vi "Array Variant to Cluster Variant.vi"(1 "Array":variant[](array[variant])) -> (0 "Cluster":variant)   [LabVIEW 2017, in "LabPack.lvlib"] (continued)
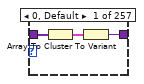
[diagram p2: hidden frame]
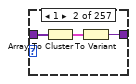
[diagram p3: hidden frame]
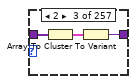
[diagram p4: hidden frame]
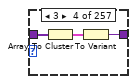
[diagram p5: hidden frame]
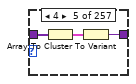
[diagram p6: hidden frame]
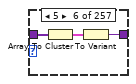
[diagram p7: hidden frame]
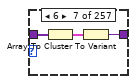
[diagram p8: hidden frame]
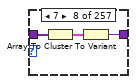
[diagram p9: hidden frame]
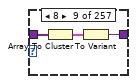
[diagram p10: hidden frame]
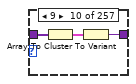
[diagram p11: hidden frame]
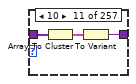
[diagram p12: hidden frame]
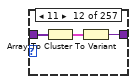
[diagram p13: hidden frame]
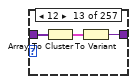
[diagram p14: hidden frame]
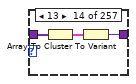
[diagram p15: hidden frame]
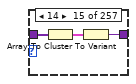
[diagram p16: hidden frame]
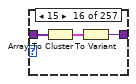
[diagram p17: hidden frame]
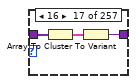
[diagram p18: hidden frame]
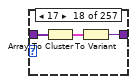
[diagram p19: hidden frame]
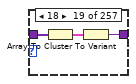
[diagram p20: hidden frame]
      n45 = Array To Cluster(array=w69) -> (cluster=w68:T19)
      n46 = To Variant(anything=w68) -> (Variant=w67:variant)
    }
    frame 22 {
      n47 = Array To Cluster(array=w72) -> (cluster=w71:T20)
      n48 = To Variant(anything=w71) -> (Variant=w70:variant)
    }
    frame 23 {
      n49 = Array To Cluster(array=w75) -> (cluster=w74:T21)
      n50 = To Variant(anything=w74) -> (Variant=w73:variant)
    }
    frame 24 {
      n51 = Array To Cluster(array=w78) -> (cluster=w77:T22)
      n52 = To Variant(anything=w77) -> (Variant=w76:variant)
    }
    frame 25 {
      n53 = Array To Cluster(array=w81) -> (cluster=w80:T23)
      n54 = To Variant(anything=w80) -> (Variant=w79:variant)
    }
    frame 26 {
      n55 = Array To Cluster(array=w84) -> (cluster=w83:T24)
      n56 = To Variant(anything=w83) -> (Variant=w82:variant)
    }
    frame 27 {
      n57 = Array To Cluster(array=w87) -> (cluster=w86:T25)
      n58 = To Variant(anything=w86) -> (Variant=w85:variant)
    }
    frame 28 {
      n59 = Array To Cluster(array=w90) -> (cluster=w89:T26)
      n60 = To Variant(anything=w89) -> (Variant=w88:variant)
    }
    frame 29 {
      n61 = Array To Cluster(array=w93) -> (cluster=w92:T27)
      n62 = To Variant(anything=w92) -> (Variant=w91:variant)
    }
    frame 30 {
      n63 = Array To Cluster(array=w96) -> (cluster=w95:T28)
      n64 = To Variant(anything=w95) -> (Variant=w94:variant)
    }
    frame 31 {
      n65 = Array To Cluster(array=w99) -> (cluster=w98:T29)
      n66 = To Variant(anything=w98) -> (Variant=w97:variant)
    }
    frame 32 {
      n67 = Array To Cluster(array=w102) -> (cluster=w101:T30)
      n68 = To Variant(anything=w101) -> (Variant=w100:variant)
    }
    frame 33 {
      n69 = Array To Cluster(array=w105) -> (cluster=w104:T31)
      n70 = To Variant(anything=w104) -> (Variant=w103:variant)
    }
    frame 34 {
      n71 = Array To Cluster(array=w108) -> (cluster=w107:T32)
      n72 = To Variant(anything=w107) -> (Variant=w106:variant)
    }
    frame 35 {
      n73 = Array To Cluster(array=w111) -> (cluster=w110:T33)
      n74 = To Variant(anything=w110) -> (Variant=w109:variant)
    }
    frame 36 {
      n75 = Array To Cluster(array=w114) -> (cluster=w113:T34)
      n76 = To Variant(anything=w113) -> (Variant=w112:variant)
    }
    frame 37 {
      n77 = Array To Cluster(array=w117) -> (cluster=w116:T35)
      n78 = To Variant(anything=w116) -> (Variant=w115:variant)
    }
    frame 38 {
      n79 = Array To Cluster(array=w120) -> (cluster=w119:T36)
      n80 = To Variant(anything=w119) -> (Variant=w118:variant)
    }
    frame 39 {
      n81 = Array To Cluster(array=w123) -> (cluster=w122:T37)
      n82 = To Variant(anything=w122) -> (Variant=w121:variant)
    }
    frame 40 {
      n83 = Array To Cluster(array=w126) -> (cluster=w125:T38)
      n84 = To Variant(anything=w125) -> (Variant=w124:variant)
    }
    frame 41 {
      n85 = Array To Cluster(array=w129) -> (cluster=w128:T39)
      n86 = To Variant(anything=w128) -> (Variant=w127:variant)
    }
    frame 42 {
      n87 = Array To Cluster(array=w132) -> (cluster=w131:T40)
      n88 = To Variant(anything=w131) -> (Variant=w130:variant)
    }
    frame 43 {
      n89 = Array To Cluster(array=w135) -> (cluster=w134:T41)
      n90 = To Variant(anything=w134) -> (Variant=w133:variant)
    }
    frame 44 {
      n91 = Array To Cluster(array=w138) -> (cluster=w137:T42)
      n92 = To Variant(anything=w137) -> (Variant=w136:variant)
    }
    frame 45 {
      n93 = Array To Cluster(array=w141) -> (cluster=w140:T43)
      n94 = To Variant(anything=w140) -> (Variant=w139:variant)
    }
    frame 46 {
      n95 = Array To Cluster(array=w144) -> (cluster=w143:T44)
      n96 = To Variant(anything=w143) -> (Variant=w142:variant)
    }
    frame 47 {
      n97 = Array To Cluster(array=w147) -> (cluster=w146:T45)
      n98 = To Variant(anything=w146) -> (Variant=w145:variant)
    }
    frame 48 {
      n99 = Array To Cluster(array=w150) -> (cluster=w149:T46)
      n100 = To Variant(anything=w149) -> (Variant=w148:variant)
    }
    frame 49 {
      n101 = Array To Cluster(array=w153) -> (cluster=w152:T47)
      n102 = To Variant(anything=w152) -> (Variant=w151:variant)
    }
    frame 50 {
      n103 = Array To Cluster(array=w156) -> (cluster=w155:T48)
      n104 = To Variant(anything=w155) -> (Variant=w154:variant)
    }
    frame 51 {
      n105 = Array To Cluster(array=w159) -> (cluster=w158:T49)
      n106 = To Variant(anything=w158) -> (Variant=w157:variant)
    }
    frame 52 {
      n107 = Array To Cluster(array=w162) -> (cluster=w161:T50)
      n108 = To Variant(anything=w161) -> (Variant=w160:variant)
    }
    frame 53 {
      n109 = Array To Cluster(array=w165) -> (cluster=w164:T51)
      n110 = To Variant(anything=w164) -> (Variant=w163:variant)
    }
    frame 54 {
      n111 = Array To Cluster(array=w168) -> (cluster=w167:T52)
      n112 = To Variant(anything=w167) -> (Variant=w166:variant)
    }
    frame 55 {
      n113 = Array To Cluster(array=w171) -> (cluster=w170:T53)
      n114 = To Variant(anything=w170) -> (Variant=w169:variant)
    }
    frame 56 {
      n115 = Array To Cluster(array=w174) -> (cluster=w173:T54)
      n116 = To Variant(anything=w173) -> (Variant=w172:variant)
    }
    frame 57 {
      n117 = Array To Cluster(array=w177) -> (cluster=w176:T55)
      n118 = To Variant(anything=w176) -> (Variant=w175:variant)
    }
    frame 58 {
      n119 = Array To Cluster(array=w180) -> (cluster=w179:T56)
      n120 = To Variant(anything=w179) -> (Variant=w178:variant)
    }
    frame 59 {
      n121 = Array To Cluster(array=w183) -> (cluster=w182:T57)
      n122 = To Variant(anything=w182) -> (Variant=w181:variant)
    }
    frame 60 {
      n123 = Array To Cluster(array=w186) -> (cluster=w185:T58)
      n124 = To Variant(anything=w185) -> (Variant=w184:variant)
    }
    frame 61 {
      n125 = Array To Cluster(array=w189) -> (cluster=w188:T59)
      n126 = To Variant(anything=w188) -> (Variant=w187:variant)
    }
    frame 62 {
      n127 = Array To Cluster(array=w192) -> (cluster=w191:T60)
      n128 = To Variant(anything=w191) -> (Variant=w190:variant)
    }
    frame 63 {
      n129 = Array To Cluster(array=w195) -> (cluster=w194:T61)
      n130 = To Variant(anything=w194) -> (Variant=w193:variant)
    }
    frame 64 {
      n131 = Array To Cluster(array=w198) -> (cluster=w197:T62)
      n132 = To Variant(anything=w197) -> (Variant=w196:variant)
    }
    frame 65 {
      n133 = Array To Cluster(array=w201) -> (cluster=w200:T63)
      n134 = To Variant(anything=w200) -> (Variant=w199:variant)
    }
    frame 66 {
      n135 = Array To Cluster(array=w204) -> (cluster=w203:T64)
      n136 = To Variant(anything=w203) -> (Variant=w202:variant)
    }
    frame 67 {
      n137 = Array To Cluster(array=w207) -> (cluster=w206:T65)
      n138 = To Variant(anything=w206) -> (Variant=w205:variant)
    }
    frame 68 {
      n139 = Array To Cluster(array=w210) -> (cluster=w209:T66)
      n140 = To Variant(anything=w209) -> (Variant=w208:variant)
    }
    frame 69 {
      n141 = Array To Cluster(array=w213) -> (cluster=w212:T67)
      n142 = To Variant(anything=w212) -> (Variant=w211:variant)
    }
    frame 70 {
      n143 = Array To Cluster(array=w216) -> (cluster=w215:T68)
      n144 = To Variant(anything=w215) -> (Variant=w214:variant)
    }
    frame 71 {
      n145 = Array To Cluster(array=w219) -> (cluster=w218:T69)
      n146 = To Variant(anything=w218) -> (Variant=w217:variant)
    }
    frame 72 {
      n147 = Array To Cluster(array=w222) -> (cluster=w221:T70)
      n148 = To Variant(anything=w221) -> (Variant=w220:variant)
    }
    frame 73 {
      n149 = Array To Cluster(array=w225) -> (cluster=w224:T71)
      n150 = To Variant(anything=w224) -> (Variant=w223:variant)
    }
    frame 74 {
      n151 = Array To Cluster(array=w228) -> (cluster=w227:T72)
      n152 = To Variant(anything=w227) -> (Variant=w226:variant)
    }
    frame 75 {
      n153 = Array To Cluster(array=w231) -> (cluster=w230:T73)
      n154 = To Variant(anything=w230) -> (Variant=w229:variant)
    }
    frame 76 {
      n155 = Array To Cluster(array=w234) -> (cluster=w233:T74)
      n156 = To Variant(anything=w233) -> (Variant=w232:variant)
    }
    frame 77 {
      n157 = Array To Cluster(array=w237) -> (cluster=w236:T75)
      n158 = To Variant(anything=w236) -> (Variant=w235:variant)
    }
    frame 78 {
      n159 = Array To Cluster(array=w240) -> (cluster=w239:T76)
      n160 = To Variant(anything=w239) -> (Variant=w238:variant)
    }
    frame 79 {
      n161 = Array To Cluster(array=w243) -> (cluster=w242:T77)
      n162 = To Variant(anything=w242) -> (Variant=w241:variant)
    }
    frame 80 {
      n163 = Array To Cluster(array=w246) -> (cluster=w245:T78)
      n164 = To Variant(anything=w245) -> (Variant=w244:variant)
    }
    frame 81 {
      n165 = Array To Cluster(array=w249) -> (cluster=w248:T79)
      n166 = To Variant(anything=w248) -> (Variant=w247:variant)
    }
    frame 82 {
      n167 = Array To Cluster(array=w252) -> (cluster=w251:T80)
      n168 = To Variant(anything=w251) -> (Variant=w250:variant)
    }
    frame 83 {
      n169 = Array To Cluster(array=w255) -> (cluster=w254:T81)
      n170 = To Variant(anything=w254) -> (Variant=w253:variant)
    }
    frame 84 {
      n171 = Array To Cluster(array=w258) -> (cluster=w257:T82)
      n172 = To Variant(anything=w257) -> (Variant=w256:variant)
    }
    frame 85 {
      n173 = Array To Cluster(array=w261) -> (cluster=w260:T83)
      n174 = To Variant(anything=w260) -> (Variant=w259:variant)
    }
    frame 86 {
      n175 = Array To Cluster(array=w264) -> (cluster=w263:T84)
      n176 = To Variant(anything=w263) -> (Variant=w262:variant)
    }
    frame 87 {
      n177 = Array To Cluster(array=w267) -> (cluster=w266:T85)
      n178 = To Variant(anything=w266) -> (Variant=w265:variant)
    }
    frame 88 {
      n179 = Array To Cluster(array=w270) -> (cluster=w269:T86)
      n180 = To Variant(anything=w269) -> (Variant=w268:variant)
    }
    frame 89 {
      n181 = Array To Cluster(array=w273) -> (cluster=w272:T87)
      n182 = To Variant(anything=w272) -> (Variant=w271:variant)
    }
    frame 90 {
      n183 = Array To Cluster(array=w276) -> (cluster=w275:T88)
      n184 = To Variant(anything=w275) -> (Variant=w274:variant)
    }
    frame 91 {
      n185 = Array To Cluster(array=w279) -> (cluster=w278:T89)
      n186 = To Variant(anything=w278) -> (Variant=w277:variant)
    }
    frame 92 {
      n187 = Array To Cluster(array=w282) -> (cluster=w281:T90)
      n188 = To Variant(anything=w281) -> (Variant=w280:variant)
    }
    frame 93 {
      n189 = Array To Cluster(array=w285) -> (cluster=w284:T91)
      n190 = To Variant(anything=w284) -> (Variant=w283:variant)
    }
    frame 94 {
      n191 = Array To Cluster(array=w288) -> (cluster=w287:T92)
      n192 = To Variant(anything=w287) -> (Variant=w286:variant)
    }
    frame 95 {
      n193 = Array To Cluster(array=w291) -> (cluster=w290:T93)
      n194 = To Variant(anything=w290) -> (Variant=w289:variant)
    }
    frame 96 {
      n195 = Array To Cluster(array=w294) -> (cluster=w293:T94)
      n196 = To Variant(anything=w293) -> (Variant=w292:variant)
    }
    frame 97 {
      n197 = Array To Cluster(array=w297) -> (cluster=w296:T95)
      n198 = To Variant(anything=w296) -> (Variant=w295:variant)
    }
    frame 98 {
      n199 = Array To Cluster(array=w300) -> (cluster=w299:T96)
      n200 = To Variant(anything=w299) -> (Variant=w298:variant)
    }
    frame 99 {
      n201 = Array To Cluster(array=w303) -> (cluster=w302:T97)
      n202 = To Variant(anything=w302) -> (Variant=w301:variant)
    }
    frame 100 {
      n203 = Array To Cluster(array=w306) -> (cluster=w305:T98)
      n204 = To Variant(anything=w305) -> (Variant=w304:variant)
    }
    frame 101 {
      n205 = Array To Cluster(array=w309) -> (cluster=w308:T99)
      n206 = To Variant(anything=w308) -> (Variant=w307:variant)
    }
    frame 102 {
      n207 = Array To Cluster(array=w312) -> (cluster=w311:T100)
      n208 = To Variant(anything=w311) -> (Variant=w310:variant)
    }
    frame 103 {
      n209 = Array To Cluster(array=w315) -> (cluster=w314:T101)
      n210 = To Variant(anything=w314) -> (Variant=w313:variant)
    }
    frame 104 {
      n211 = Array To Cluster(array=w318) -> (cluster=w317:T102)
      n212 = To Variant(anything=w317) -> (Variant=w316:variant)
    }
    frame 105 {
      n213 = Array To Cluster(array=w321) -> (cluster=w320:T103)
      n214 = To Variant(anything=w320) -> (Variant=w319:variant)
    }
    frame 106 {
      n215 = Array To Cluster(array=w324) -> (cluster=w323:T104)
      n216 = To Variant(anything=w323) -> (Variant=w322:variant)
    }
    frame 107 {
      n217 = Array To Cluster(array=w327) -> (cluster=w326:T105)
      n218 = To Variant(anything=w326) -> (Variant=w325:variant)
    }
    frame 108 {
      n219 = Array To Cluster(array=w330) -> (cluster=w329:T106)
      n220 = To Variant(anything=w329) -> (Variant=w328:variant)
    }
    frame 109 {
      n221 = Array To Cluster(array=w333) -> (cluster=w332:T107)
      n222 = To Variant(anything=w332) -> (Variant=w331:variant)
    }
    frame 110 {
      n223 = Array To Cluster(array=w336) -> (cluster=w335:T108)
      n224 = To Variant(anything=w335) -> (Variant=w334:variant)
    }
    frame 111 {
      n225 = Array To Cluster(array=w339) -> (cluster=w338:T109)
      n226 = To Variant(anything=w338) -> (Variant=w337:variant)
    }
    frame 112 {
      n227 = Array To Cluster(array=w342) -> (cluster=w341:T110)
      n228 = To Variant(anything=w341) -> (Variant=w340:variant)
    }
    frame 113 {
      n229 = Array To Cluster(array=w345) -> (cluster=w344:T111)
      n230 = To Variant(anything=w344) -> (Variant=w343:variant)
    }
    frame 114 {
      n231 = Array To Cluster(array=w348) -> (cluster=w347:T112)
      n232 = To Variant(anything=w347) -> (Variant=w346:variant)
    }
    frame 115 {
      n233 = Array To Cluster(array=w351) -> (cluster=w350:T113)
      n234 = To Variant(anything=w350) -> (Variant=w349:variant)
    }
    frame 116 {
      n235 = Array To Cluster(array=w354) -> (cluster=w353:T114)
      n236 = To Variant(anything=w353) -> (Variant=w352:variant)
    }
    frame 117 {
      n237 = Array To Cluster(array=w357) -> (cluster=w356:T115)
      n238 = To Variant(anything=w356) -> (Variant=w355:variant)
    }
    frame 118 {
      n239 = Array To Cluster(array=w360) -> (cluster=w359:T116)
      n240 = To Variant(anything=w359) -> (Variant=w358:variant)
    }
    frame 119 {
      n241 = Array To Cluster(array=w363) -> (cluster=w362:T117)
      n242 = To Variant(anything=w362) -> (Variant=w361:variant)
    }
    frame 120 {
      n243 = Array To Cluster(array=w366) -> (cluster=w365:T118)
      n244 = To Variant(anything=w365) -> (Variant=w364:variant)
    }
    frame 121 {
      n245 = Array To Cluster(array=w369) -> (cluster=w368:T119)
      n246 = To Variant(anything=w368) -> (Variant=w367:variant)
    }
    frame 122 {
      n247 = Array To Cluster(array=w372) -> (cluster=w371:T120)
      n248 = To Variant(anything=w371) -> (Variant=w370:variant)
    }
    frame 123 {
      n249 = Array To Cluster(array=w375) -> (cluster=w374:T121)
      n250 = To Variant(anything=w374) -> (Variant=w373:variant)
    }
    frame 124 {
      n251 = Array To Cluster(array=w378) -> (cluster=w377:T122)
      n252 = To Variant(anything=w377) -> (Variant=w376:variant)
    }
    frame 125 {
      n253 = Array To Cluster(array=w381) -> (cluster=w380:T123)
      n254 = To Variant(anything=w380) -> (Variant=w379:variant)
    }
    frame 126 {
      n255 = Array To Cluster(array=w384) -> (cluster=w383:T124)
      n256 = To Variant(anything=w383) -> (Variant=w382:variant)
    }
    frame 127 {
      n257 = Array To Cluster(array=w387) -> (cluster=w386:T125)
      n258 = To Variant(anything=w386) -> (Variant=w385:variant)
    }
    frame 128 {
      n259 = Array To Cluster(array=w390) -> (cluster=w389:T126)
      n260 = To Variant(anything=w389) -> (Variant=w388:variant)
    }
    frame 129 {
      n261 = Array To Cluster(array=w393) -> (cluster=w392:T127)
      n262 = To Variant(anything=w392) -> (Variant=w391:variant)
    }
    frame 130 {
      n263 = Array To Cluster(array=w396) -> (cluster=w395:T128)
      n264 = To Variant(anything=w395) -> (Variant=w394:variant)
    }
    frame 131 {
      n265 = Array To Cluster(array=w399) -> (cluster=w398:T129)
      n266 = To Variant(anything=w398) -> (Variant=w397:variant)
    }
    frame 132 {
      n267 = Array To Cluster(array=w402) -> (cluster=w401:T130)
      n268 = To Variant(anything=w401) -> (Variant=w400:variant)
    }
    frame 133 {
      n269 = Array To Cluster(array=w405) -> (cluster=w404:T131)
      n270 = To Variant(anything=w404) -> (Variant=w403:variant)
    }
    frame 134 {
      n271 = Array To Cluster(array=w408) -> (cluster=w407:T132)
      n272 = To Variant(anything=w407) -> (Variant=w406:variant)
    }
    frame 135 {
      n273 = Array To Cluster(array=w411) -> (cluster=w410:T133)
      n274 = To Variant(anything=w410) -> (Variant=w409:variant)
    }
    frame 136 {
      n275 = Array To Cluster(array=w414) -> (cluster=w413:T134)
      n276 = To Variant(anything=w413) -> (Variant=w412:variant)
    }
    frame 137 {
      n277 = Array To Cluster(array=w417) -> (cluster=w416:T135)
      n278 = To Variant(anything=w416) -> (Variant=w415:variant)
    }
    frame 138 {
      n279 = Array To Cluster(array=w420) -> (cluster=w419:T136)
      n280 = To Variant(anything=w419) -> (Variant=w418:variant)
    }
    frame 139 {
      n281 = Array To Cluster(array=w423) -> (cluster=w422:T137)
      n282 = To Variant(anything=w422) -> (Variant=w421:variant)
    }
    frame 140 {
      n283 = Array To Cluster(array=w426) -> (cluster=w425:T138)
      n284 = To Variant(anything=w425) -> (Variant=w424:variant)
    }
    frame 141 {
      n285 = Array To Cluster(array=w429) -> (cluster=w428:T139)
      n286 = To Variant(anything=w428) -> (Variant=w427:variant)
    }
    frame 142 {
      n287 = Array To Cluster(array=w432) -> (cluster=w431:T140)
      n288 = To Variant(anything=w431) -> (Variant=w430:variant)
    }
    frame 143 {
      n289 = Array To Cluster(array=w435) -> (cluster=w434:T141)
      n290 = To Variant(anything=w434) -> (Variant=w433:variant)
    }
    frame 144 {
      n291 = Array To Cluster(array=w438) -> (cluster=w437:T142)
      n292 = To Variant(anything=w437) -> (Variant=w436:variant)
    }
    frame 145 {
      n293 = Array To Cluster(array=w441) -> (cluster=w440:T143)
      n294 = To Variant(anything=w440) -> (Variant=w439:variant)
    }
    frame 146 {
      n295 = Array To Cluster(array=w444) -> (cluster=w443:T144)
      n296 = To Variant(anything=w443) -> (Variant=w442:variant)
    }
    frame 147 {
      n297 = Array To Cluster(array=w447) -> (cluster=w446:T145)
      n298 = To Variant(anything=w446) -> (Variant=w445:variant)
    }
    frame 148 {
      n299 = Array To Cluster(array=w450) -> (cluster=w449:T146)
      n300 = To Variant(anything=w449) -> (Variant=w448:variant)
    }
    frame 149 {
      n301 = Array To Cluster(array=w453) -> (cluster=w452:T147)
      n302 = To Variant(anything=w452) -> (Variant=w451:variant)
    }
    frame 150 {
      n303 = Array To Cluster(array=w456) -> (cluster=w455:T148)
      n304 = To Variant(anything=w455) -> (Variant=w454:variant)
    }
    frame 151 {
      n305 = Array To Cluster(array=w459) -> (cluster=w458:T149)
      n306 = To Variant(anything=w458) -> (Variant=w457:variant)
    }
    frame 152 {
      n307 = Array To Cluster(array=w462) -> (cluster=w461:T150)
      n308 = To Variant(anything=w461) -> (Variant=w460:variant)
    }
    frame 153 {
      n309 = Array To Cluster(array=w465) -> (cluster=w464:T151)
      n310 = To Variant(anything=w464) -> (Variant=w463:variant)
    }
    frame 154 {
      n311 = Array To Cluster(array=w468) -> (cluster=w467:T152)
      n312 = To Variant(anything=w467) -> (Variant=w466:variant)
    }
    frame 155 {
      n313 = Array To Cluster(array=w471) -> (cluster=w470:T153)
      n314 = To Variant(anything=w470) -> (Variant=w469:variant)
    }
    frame 156 {
      n315 = Array To Cluster(array=w474) -> (cluster=w473:T154)
      n316 = To Variant(anything=w473) -> (Variant=w472:variant)
    }
    frame 157 {
      n317 = Array To Cluster(array=w477) -> (cluster=w476:T155)
      n318 = To Variant(anything=w476) -> (Variant=w475:variant)
    }
    frame 158 {
      n319 = Array To Cluster(array=w480) -> (cluster=w479:T156)
      n320 = To Variant(anything=w479) -> (Variant=w478:variant)
    }
    frame 159 {
      n321 = Array To Cluster(array=w483) -> (cluster=w482:T157)
      n322 = To Variant(anything=w482) -> (Variant=w481:variant)
    }
    frame 160 {
      n323 = Array To Cluster(array=w486) -> (cluster=w485:T158)
      n324 = To Variant(anything=w485) -> (Variant=w484:variant)
    }
    frame 161 {
      n325 = Array To Cluster(array=w489) -> (cluster=w488:T159)
      n326 = To Variant(anything=w488) -> (Variant=w487:variant)
    }
    frame 162 {
      n327 = Array To Cluster(array=w492) -> (cluster=w491:T160)
      n328 = To Variant(anything=w491) -> (Variant=w490:variant)
    }
    frame 163 {
      n329 = Array To Cluster(array=w495) -> (cluster=w494:T161)
      n330 = To Variant(anything=w494) -> (Variant=w493:variant)
    }
    frame 164 {
      n331 = Array To Cluster(array=w498) -> (cluster=w497:T162)
      n332 = To Variant(anything=w497) -> (Variant=w496:variant)
    }
    frame 165 {
      n333 = Array To Cluster(array=w501) -> (cluster=w500:T163)
      n334 = To Variant(anything=w500) -> (Variant=w499:variant)
    }
    frame 166 {
      n335 = Array To Cluster(array=w504) -> (cluster=w503:T164)
      n336 = To Variant(anything=w503) -> (Variant=w502:variant)
    }
    frame 167 {
      n337 = Array To Cluster(array=w507) -> (cluster=w506:T165)
      n338 = To Variant(anything=w506) -> (Variant=w505:variant)
    }
    frame 168 {
      n339 = Array To Cluster(array=w510) -> (cluster=w509:T166)
      n340 = To Variant(anything=w509) -> (Variant=w508:variant)
    }
    frame 169 {
      n341 = Array To Cluster(array=w513) -> (cluster=w512:T167)
      n342 = To Variant(anything=w512) -> (Variant=w511:variant)
    }
    frame 170 {
      n343 = Array To Cluster(array=w516) -> (cluster=w515:T168)
      n344 = To Variant(anything=w515) -> (Variant=w514:variant)
    }
    frame 171 {
      n345 = Array To Cluster(array=w519) -> (cluster=w518:T169)
      n346 = To Variant(anything=w518) -> (Variant=w517:variant)
    }
    frame 172 {
      n347 = Array To Cluster(array=w522) -> (cluster=w521:T170)
      n348 = To Variant(anything=w521) -> (Variant=w520:variant)
    }
    frame 173 {
      n349 = Array To Cluster(array=w525) -> (cluster=w524:T171)
      n350 = To Variant(anything=w524) -> (Variant=w523:variant)
    }
    frame 174 {
      n351 = Array To Cluster(array=w528) -> (cluster=w527:T172)
      n352 = To Variant(anything=w527) -> (Variant=w526:variant)
    }
    frame 175 {
      n353 = Array To Cluster(array=w531) -> (cluster=w530:T173)
      n354 = To Variant(anything=w530) -> (Variant=w529:variant)
    }
    frame 176 {
      n355 = Array To Cluster(array=w534) -> (cluster=w533:T174)
      n356 = To Variant(anything=w533) -> (Variant=w532:variant)
    }
    frame 177 {
      n357 = Array To Cluster(array=w537) -> (cluster=w536:T175)
      n358 = To Variant(anything=w536) -> (Variant=w535:variant)
    }
    frame 178 {
      n359 = Array To Cluster(array=w540) -> (cluster=w539:T176)
      n360 = To Variant(anything=w539) -> (Variant=w538:variant)
    }
    frame 179 {
      n361 = Array To Cluster(array=w543) -> (cluster=w542:T177)
      n362 = To Variant(anything=w542) -> (Variant=w541:variant)
    }
    frame 180 {
      n363 = Array To Cluster(array=w546) -> (cluster=w545:T178)
      n364 = To Variant(anything=w545) -> (Variant=w544:variant)
    }
    frame 181 {
      n365 = Array To Cluster(array=w549) -> (cluster=w548:T179)
      n366 = To Variant(anything=w548) -> (Variant=w547:variant)
    }
    frame 182 {
      n367 = Array To Cluster(array=w552) -> (cluster=w551:T180)
      n368 = To Variant(anything=w551) -> (Variant=w550:variant)
    }
    frame 183 {
      n369 = Array To Cluster(array=w555) -> (cluster=w554:T181)
      n370 = To Variant(anything=w554) -> (Variant=w553:variant)
    }
    frame 184 {
      n371 = Array To Cluster(array=w558) -> (cluster=w557:T182)
      n372 = To Variant(anything=w557) -> (Variant=w556:variant)
    }
    frame 185 {
      n373 = Array To Cluster(array=w561) -> (cluster=w560:T183)
      n374 = To Variant(anything=w560) -> (Variant=w559:variant)
    }
    frame 186 {
      n375 = Array To Cluster(array=w564) -> (cluster=w563:T184)
      n376 = To Variant(anything=w563) -> (Variant=w562:variant)
    }
    frame 187 {
      n377 = Array To Cluster(array=w567) -> (cluster=w566:T185)
      n378 = To Variant(anything=w566) -> (Variant=w565:variant)
    }
    frame 188 {
      n379 = Array To Cluster(array=w570) -> (cluster=w569:T186)
      n380 = To Variant(anything=w569) -> (Variant=w568:variant)
    }
    frame 189 {
      n381 = Array To Cluster(array=w573) -> (cluster=w572:T187)
      n382 = To Variant(anything=w572) -> (Variant=w571:variant)
    }
    frame 190 {
      n383 = Array To Cluster(array=w576) -> (cluster=w575:T188)
      n384 = To Variant(anything=w575) -> (Variant=w574:variant)
    }
    frame 191 {
      n385 = Array To Cluster(array=w579) -> (cluster=w578:T189)
      n386 = To Variant(anything=w578) -> (Variant=w577:variant)
    }
    frame 192 {
      n387 = Array To Cluster(array=w582) -> (cluster=w581:T190)
      n388 = To Variant(anything=w581) -> (Variant=w580:variant)
    }
    frame 193 {
      n389 = Array To Cluster(array=w585) -> (cluster=w584:T191)
      n390 = To Variant(anything=w584) -> (Variant=w583:variant)
    }
    frame 194 {
      n391 = Array To Cluster(array=w588) -> (cluster=w587:T192)
      n392 = To Variant(anything=w587) -> (Variant=w586:variant)
    }
    frame 195 {
      n393 = Array To Cluster(array=w591) -> (cluster=w590:T193)
      n394 = To Variant(anything=w590) -> (Variant=w589:variant)
    }
    frame 196 {
      n395 = Array To Cluster(array=w594) -> (cluster=w593:T194)
      n396 = To Variant(anything=w593) -> (Variant=w592:variant)
    }
    frame 197 {
      n397 = Array To Cluster(array=w597) -> (cluster=w596:T195)
      n398 = To Variant(anything=w596) -> (Variant=w595:variant)
    }
    frame 198 {
      n399 = Array To Cluster(array=w600) -> (cluster=w599:T196)
      n400 = To Variant(anything=w599) -> (Variant=w598:variant)
    }
    frame 199 {
      n401 = Array To Cluster(array=w603) -> (cluster=w602:T197)
      n402 = To Variant(anything=w602) -> (Variant=w601:variant)
    }
    frame 200 {
      n403 = Array To Cluster(array=w606) -> (cluster=w605:T198)
      n404 = To Variant(anything=w605) -> (Variant=w604:variant)
    }
    frame 201 {
      n405 = Array To Cluster(array=w609) -> (cluster=w608:T199)
      n406 = To Variant(anything=w608) -> (Variant=w607:variant)
    }
    frame 202 {
      n407 = Array To Cluster(array=w612) -> (cluster=w611:T200)
      n408 = To Variant(anything=w611) -> (Variant=w610:variant)
    }
    frame 203 {
      n409 = Array To Cluster(array=w615) -> (cluster=w614:T201)
      n410 = To Variant(anything=w614) -> (Variant=w613:variant)
    }
    frame 204 {
      n411 = Array To Cluster(array=w618) -> (cluster=w617:T202)
      n412 = To Variant(anything=w617) -> (Variant=w616:variant)
    }
    frame 205 {
      n413 = Array To Cluster(array=w621) -> (cluster=w620:T203)
      n414 = To Variant(anything=w620) -> (Variant=w619:variant)
    }
    frame 206 {
      n415 = Array To Cluster(array=w624) -> (cluster=w623:T204)
      n416 = To Variant(anything=w623) -> (Variant=w622:variant)
    }
    frame 207 {
      n417 = Array To Cluster(array=w627) -> (cluster=w626:T205)
      n418 = To Variant(anything=w626) -> (Variant=w625:variant)
    }
    frame 208 {
      n419 = Array To Cluster(array=w630) -> (cluster=w629:T206)
      n420 = To Variant(anything=w629) -> (Variant=w628:variant)
    }
    frame 209 {
      n421 = Array To Cluster(array=w633) -> (cluster=w632:T207)
      n422 = To Variant(anything=w632) -> (Variant=w631:variant)
    }
    frame 210 {
      n423 = Array To Cluster(array=w636) -> (cluster=w635:T208)
      n424 = To Variant(anything=w635) -> (Variant=w634:variant)
    }
    frame 211 {
      n425 = Array To Cluster(array=w639) -> (cluster=w638:T209)
      n426 = To Variant(anything=w638) -> (Variant=w637:variant)
    }
    frame 212 {
      n427 = Array To Cluster(array=w642) -> (cluster=w641:T210)
      n428 = To Variant(anything=w641) -> (Variant=w640:variant)
    }
    frame 213 {
      n429 = Array To Cluster(array=w645) -> (cluster=w644:T211)
      n430 = To Variant(anything=w644) -> (Variant=w643:variant)
    }
    frame 214 {
      n431 = Array To Cluster(array=w648) -> (cluster=w647:T212)
      n432 = To Variant(anything=w647) -> (Variant=w646:variant)
    }
    frame 215 {
      n433 = Array To Cluster(array=w651) -> (cluster=w650:T213)
      n434 = To Variant(anything=w650) -> (Variant=w649:variant)
    }
    frame 216 {
      n435 = Array To Cluster(array=w654) -> (cluster=w653:T214)
      n436 = To Variant(anything=w653) -> (Variant=w652:variant)
    }
    frame 217 {
      n437 = Array To Cluster(array=w657) -> (cluster=w656:T215)
      n438 = To Variant(anything=w656) -> (Variant=w655:variant)
    }
    frame 218 {
      n439 = Array To Cluster(array=w660) -> (cluster=w659:T216)
      n440 = To Variant(anything=w659) -> (Variant=w658:variant)
    }
    frame 219 {
      n441 = Array To Cluster(array=w663) -> (cluster=w662:T217)
      n442 = To Variant(anything=w662) -> (Variant=w661:variant)
    }
    frame 220 {
      n443 = Array To Cluster(array=w666) -> (cluster=w665:T218)
      n444 = To Variant(anything=w665) -> (Variant=w664:variant)
    }
    frame 221 {
      n445 = Array To Cluster(array=w669) -> (cluster=w668:T219)
      n446 = To Variant(anything=w668) -> (Variant=w667:variant)
    }
    frame 222 {
      n447 = Array To Cluster(array=w672) -> (cluster=w671:T220)
      n448 = To Variant(anything=w671) -> (Variant=w670:variant)
    }
    frame 223 {
      n449 = Array To Cluster(array=w675) -> (cluster=w674:T221)
      n450 = To Variant(anything=w674) -> (Variant=w673:variant)
    }
    frame 224 {
      n451 = Array To Cluster(array=w678) -> (cluster=w677:T222)
      n452 = To Variant(anything=w677) -> (Variant=w676:variant)
    }
    frame 225 {
      n453 = Array To Cluster(array=w681) -> (cluster=w680:T223)
      n454 = To Variant(anything=w680) -> (Variant=w679:variant)
    }
    frame 226 {
      n455 = Array To Cluster(array=w684) -> (cluster=w683:T224)
      n456 = To Variant(anything=w683) -> (Variant=w682:variant)
    }
    frame 227 {
      n457 = Array To Cluster(array=w687) -> (cluster=w686:T225)
      n458 = To Variant(anything=w686) -> (Variant=w685:variant)
    }
    frame 228 {
      n459 = Array To Cluster(array=w690) -> (cluster=w689:T226)
      n460 = To Variant(anything=w689) -> (Variant=w688:variant)
    }
    frame 229 {
      n461 = Array To Cluster(array=w693) -> (cluster=w692:T227)
      n462 = To Variant(anything=w692) -> (Variant=w691:variant)
    }
    frame 230 {
      n463 = Array To Cluster(array=w696) -> (cluster=w695:T228)
      n464 = To Variant(anything=w695) -> (Variant=w694:variant)
    }
    frame 231 {
      n465 = Array To Cluster(array=w699) -> (cluster=w698:T229)
      n466 = To Variant(anything=w698) -> (Variant=w697:variant)
    }
    frame 232 {
      n467 = Array To Cluster(array=w702) -> (cluster=w701:T230)
      n468 = To Variant(anything=w701) -> (Variant=w700:variant)
    }
    frame 233 {
      n469 = Array To Cluster(array=w705) -> (cluster=w704:T231)
      n470 = To Variant(anything=w704) -> (Variant=w703:variant)
    }
    frame 234 {
      n471 = Array To Cluster(array=w708) -> (cluster=w707:T232)
      n472 = To Variant(anything=w707) -> (Variant=w706:variant)
    }
    frame 235 {
      n473 = Array To Cluster(array=w711) -> (cluster=w710:T233)
      n474 = To Variant(anything=w710) -> (Variant=w709:variant)
    }
    frame 236 {
      n475 = Array To Cluster(array=w714) -> (cluster=w713:T234)
      n476 = To Variant(anything=w713) -> (Variant=w712:variant)
    }
    frame 237 {
      n477 = Array To Cluster(array=w717) -> (cluster=w716:T235)
      n478 = To Variant(anything=w716) -> (Variant=w715:variant)
    }
    frame 238 {
      n479 = Array To Cluster(array=w720) -> (cluster=w719:T236)
      n480 = To Variant(anything=w719) -> (Variant=w718:variant)
    }
    frame 239 {
      n481 = Array To Cluster(array=w723) -> (cluster=w722:T237)
      n482 = To Variant(anything=w722) -> (Variant=w721:variant)
    }
    frame 240 {
      n483 = Array To Cluster(array=w726) -> (cluster=w725:T238)
      n484 = To Variant(anything=w725) -> (Variant=w724:variant)
    }
    frame 241 {
      n485 = Array To Cluster(array=w729) -> (cluster=w728:T239)
      n486 = To Variant(anything=w728) -> (Variant=w727:variant)
    }
    frame 242 {
      n487 = Array To Cluster(array=w732) -> (cluster=w731:T240)
      n488 = To Variant(anything=w731) -> (Variant=w730:variant)
    }
    frame 243 {
      n489 = Array To Cluster(array=w735) -> (cluster=w734:T241)
      n490 = To Variant(anything=w734) -> (Variant=w733:variant)
    }
    frame 244 {
      n491 = Array To Cluster(array=w738) -> (cluster=w737:T242)
      n492 = To Variant(anything=w737) -> (Variant=w736:variant)
    }
    frame 245 {
      n493 = Array To Cluster(array=w741) -> (cluster=w740:T243)
      n494 = To Variant(anything=w740) -> (Variant=w739:variant)
    }
    frame 246 {
      n495 = Array To Cluster(array=w744) -> (cluster=w743:T244)
      n496 = To Variant(anything=w743) -> (Variant=w742:variant)
    }
    frame 247 {
      n497 = Array To Cluster(array=w747) -> (cluster=w746:T245)
      n498 = To Variant(anything=w746) -> (Variant=w745:variant)
    }
    frame 248 {
      n499 = Array To Cluster(array=w750) -> (cluster=w749:T246)
      n500 = To Variant(anything=w749) -> (Variant=w748:variant)
    }
    frame 249 {
      n501 = Array To Cluster(array=w753) -> (cluster=w752:T247)
      n502 = To Variant(anything=w752) -> (Variant=w751:variant)
    }
    frame 250 {
      n503 = Array To Cluster(array=w756) -> (cluster=w755:T248)
      n504 = To Variant(anything=w755) -> (Variant=w754:variant)
    }
    frame 251 {
      n505 = Array To Cluster(array=w759) -> (cluster=w758:T249)
      n506 = To Variant(anything=w758) -> (Variant=w757:variant)
    }
    frame 252 {
      n507 = Array To Cluster(array=w762) -> (cluster=w761:T250)
      n508 = To Variant(anything=w761) -> (Variant=w760:variant)
    }
    frame 253 {
      n509 = Array To Cluster(array=w765) -> (cluster=w764:T251)
      n510 = To Variant(anything=w764) -> (Variant=w763:variant)
    }
    frame 254 {
      n511 = Array To Cluster(array=w768) -> (cluster=w767:T252)
      n512 = To Variant(anything=w767) -> (Variant=w766:variant)
    }
    frame 255 {
      n513 = Array To Cluster(array=w771) -> (cluster=w770:T253)
      n514 = To Variant(anything=w770) -> (Variant=w769:variant)
    }
    frame 256 {
      n515 = Array To Cluster(array=w774) -> (cluster=w773:T254)
      n516 = To Variant(anything=w773) -> (Variant=w772:variant)
    }
  }
  "Cluster" <- w1
